vi "comm open.vi"(4 "error in (no error)":errorcluster, 6 "open duplicate?":bool, 7 "Comm Port Name":string) -> (0 "error out":errorcluster, 3 "Comm Handle":u64)   [LabVIEW 2009, in "lvserial.lvlib"]
doc: "Opens the serial port. If the duplicate value is true, only a duplicate of the serial port will be opened (if the serial port is already open)."
uses:
  lvserial.lvlib
  x64/Release/lvserial.dll
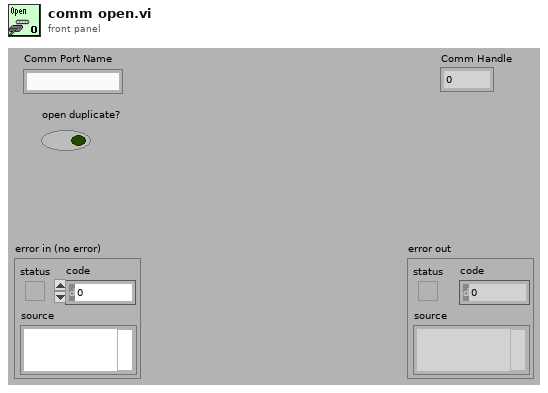
[diagram p1: front panel]
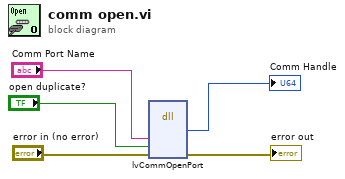
[diagram p0: block diagram]
diagram:
  n1 = dll-call lib="C:/Users/Admin/Desktop/lvserial_source_1-2-13/x64/Release/lvserial.dll" fn="lvCommOpenPort"("port"="Comm Port Name", "fDuplicate"="open duplicate?", "error"="error in (no error)") -> ("phComm"=→"Comm Handle":u64, "error"=→"error out":errorcluster)  [unwired: 5 in, 4 out]
